vi "ConfigureLinkButton.vi"(8 "Position:Left":i32, 9 "is section header?":bool, 10 "GettingStartedWindow.lvlib:ClickableText.lvclass":refnum<class "ClickableText.lvclass">, 11 "Link Button 1":refnum<vi>) -> (2 "Top":i32, 3 "Link Button 2":refnum<vi>)   [LabVIEW 2009, in "NavScreen.lvlib"]
uses:
  NavScreen.lvlib
  Classes/ClickableText/ClickableText.lvclass
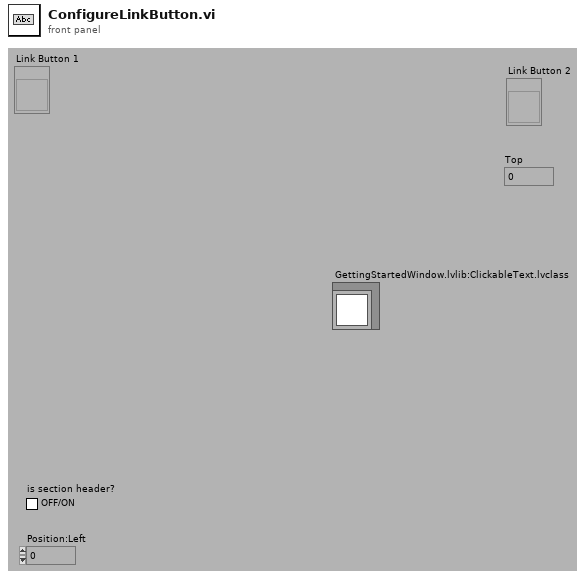
[diagram p1: front panel]
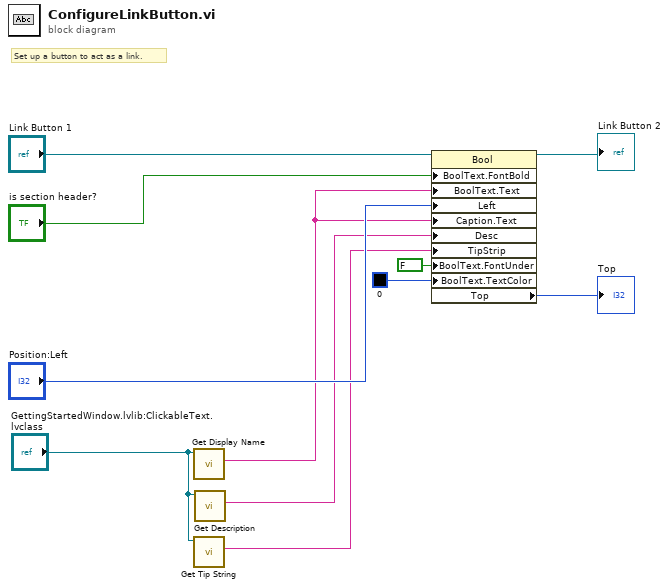
[diagram p0: block diagram]
diagram:
  # "Set up a button to act as a link."
  n1 = call-dynamic "Get Display Name.vi"("ClickableText in"="GettingStartedWindow.lvlib:ClickableText.lvclass") -> ("localized name"=w4:string)  [unwired: 8 in, 2 out]
  n2 = call "Get Tip String.vi"("ClickableText in"="GettingStartedWindow.lvlib:ClickableText.lvclass") -> ("tip string"=w1:string)  [unwired: 8 in, 2 out]
  n3 = call "Get Description.vi"("ClickableText in"="GettingStartedWindow.lvlib:ClickableText.lvclass") -> ("description"=w3:string)  [unwired: 8 in, 2 out]
  n4 = property class="Bool"(reference="Link Button 1", "BoolText.FontBold"="is section header?", "BoolText.Text"=w4, "Left"="Position:Left", "Caption.Text"=w4, "Desc"=w3, "TipStrip"=w1, "BoolText.FontUnder"=FALSE ("Boolean Text.Font:Underline"), "BoolText.TextColor"=u32 0) -> (reference out=→"Link Button 2":refnum<vi>, "Top"=→"Top":i32)  [unwired: 1 in, 1 out]
